vi "rename tag.vi"(8 "error in":errorcluster, 9 "new tag name":string, 10 "current tag name":string, 11 "tag collection in":refnum<class "tag collection.lvclass">) -> (0 "error out":errorcluster, 3 "tag collection out":refnum<class "tag collection.lvclass">)   [LabVIEW 2013, in "tag bus.lvlib" / "tag collection.lvclass"]
uses:
  tag collection.lvclass
  tag collection.lvclass/tag collection.ctl
  tag/tag descriptor.lvclass/tag descriptor.ctl
  tag/read tag name.vi
  tag bus.lvlib
  tag/tag descriptor.lvclass
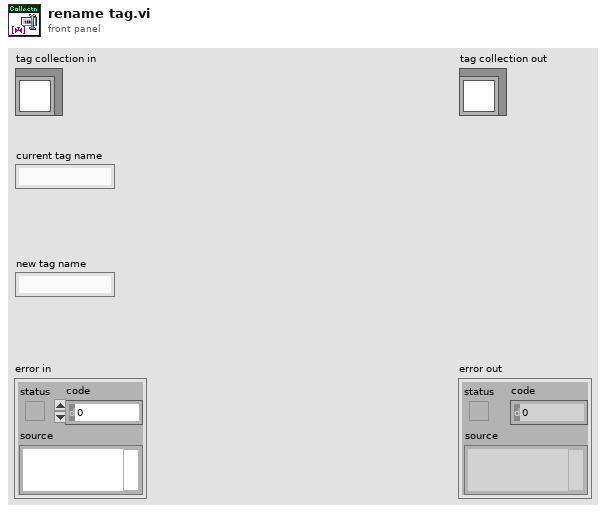
[diagram p1: front panel]
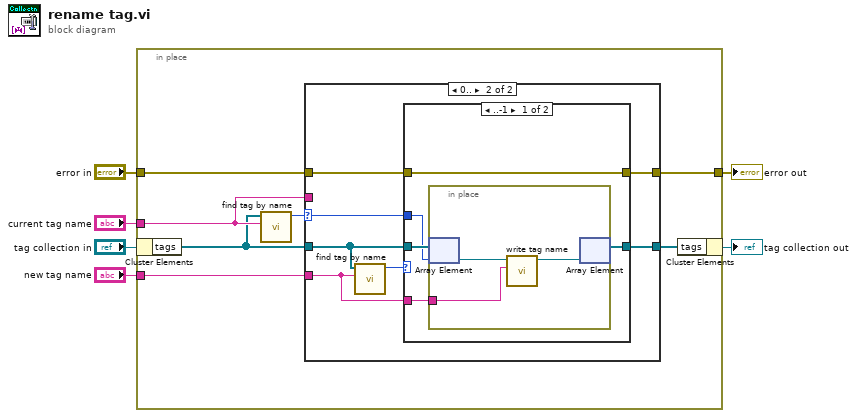
[diagram p0: block diagram]
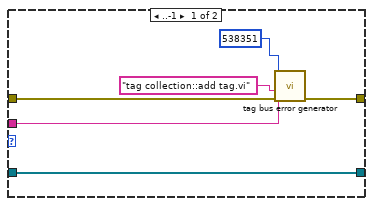
[diagram p2: hidden frame]
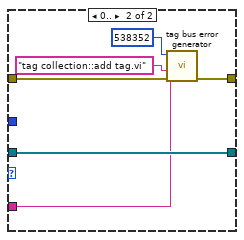
[diagram p3: hidden frame]
diagram:
  n1 = in-place {
    in-place-border: "error in" -> [w12]
    in-place-border: [w13] -> w3
    in-place-border: "current tag name" -> [w9]
    in-place-border: "new tag name" -> [w7]
    n2 = in-place-cluster #1("tag collection in") -> ("tags"=w8:refnum<class "tag descriptor.lvclass">[])
    n3 = call "find tag by name.vi"("name"=w9, "tags in"=w8) -> ("index"=w10:i32)  [unwired: 9 in]
    n4 = case shown="0.." w10 {
      selector: w10 -> [_ w21]
      tunnel: [w17 w23] -> w13
      tunnel: w12 -> [w18 w22]
      tunnel: w8 -> [w19 w24]
      tunnel: [w19 w25] -> w11
      tunnel: w9 -> [w14 _]
      tunnel: w7 -> [_ w20]
      frame ..-1 {
        n5 = call "tag bus error generator.vi"("error in"=w18, "source"="tag collection::add tag.vi", "append error message"=w14, "error code (0)"=538351) -> ("error out"=w17:errorcluster)  [unwired: 5 in]
      }
      frame 0.. {
        n6 = call "find tag by name.vi"("name"=w20, "tags in"=w24) -> ("index"=w26:i32)  [unwired: 9 in]
        n7 = case shown="..-1" w26 {
          tunnel: [w29 w40] -> w25
          tunnel: w24 -> [w30 w40]
          tunnel: [w31 w37] -> w23
          tunnel: w22 -> [w31 w36]
          tunnel: w21 -> [w28 _]
          tunnel: w20 -> [w27 w35]
          frame ..-1 {
            n8 = in-place {
              in-place-border: w27 -> [w32]
              n9 = in-place-array #2(w30, w28) -> (w34:refnum<class "tag descriptor.lvclass">)
              n10 = call "write tag name.vi"("name"=w32, "system tag in"=w34) -> ("system tag out"=w33:refnum<class "tag descriptor.lvclass">)  [unwired: 8 in, 1 out]
              n11 = in-place-array #2(w33) -> (w29:refnum<class "tag descriptor.lvclass">[])  [unwired: 1 out]
            }
          }
          frame 0.. {
            n12 = call "tag bus error generator.vi"("error in"=w36, "source"="tag collection::add tag.vi", "append error message"=w35, "error code (0)"=538352) -> ("error out"=w37:errorcluster)  [unwired: 5 in]
          }
        }
      }
    }
    n13 = in-place-cluster #1("tags"=w11) -> (→"tag collection out":refnum<class "tag collection.lvclass">)
  }
  "error out" <- w3
